vi "Initialize Hardware References.vi"(8 "error in (no error)":errorcluster caption="错误输入（无错误）", 11 "Hardware Resources in":T1={"PLC设置"={"端口选择"="COM3", "波特率"=0, "校检"=0, "数据位"=0}, "动作设置"={"自动跳法测试动作"={"夹紧"={"PLC指令"={"变量类型"=2, "PLC地址"="0", "16位/32位"=0, "写入数据(写入时有效)"=""}}, "分中"={}, "通油"={"打开主阀"={"变量类型"=2, "PLC地址"="0", "16位/32位"=0, "写入数据(写入时有效)"=""}, "打开电磁阀"={"变量类型"=2, "PLC地址"="0", "16位/32位"=0, "写入数据(写入时有效)"=""}}, "自动对中"={}, "内泄漏测试"={}, "压销"={"PLC指令"={"变量类型"=2, "PLC地址"="0", "16位/32位"=0, "写入数据(写入时有效)"=""}}}}} caption="硬件资源输入" {"动作设置"."自动跳法测试动作"."压销"."PLC指令"."16位/32位" items=["16bit", "32bit"]; "动作设置"."自动跳法测试动作"."压销"."PLC指令"."变量类型" items=["X", "Y", "M", "D"]; "动作设置"."自动跳法测试动作"."通油"."打开电磁阀"."16位/32位" items=["16bit", "32bit"]; "动作设置"."自动跳法测试动作"."通油"."打开电磁阀"."变量类型" items=["X", "Y", "M", "D"]; "动作设置"."自动跳法测试动作"."通油"."打开主阀"."16位/32位" items=["16bit", "32bit"]; "动作设置"."自动跳法测试动作"."通油"."打开主阀"."变量类型" items=["X", "Y", "M", "D"]; "动作设置"."自动跳法测试动作"."夹紧"."PLC指令"."16位/32位" items=["16bit", "32bit"]; "动作设置"."自动跳法测试动作"."夹紧"."PLC指令"."变量类型" items=["X", "Y", "M", "D"]; "PLC设置"."数据位" items=["7"=7, "8"=8]; "PLC设置"."校检" items=["无", "偶", "奇"]; "PLC设置"."波特率" items=["9600"=9600, "19200"=19200, "115200"=115200]}) -> (0 "error out":errorcluster caption="错误输出", 3 "Hardware Resources out":T1={"PLC设置"={"端口选择"="COM3", "波特率"=0, "校检"=0, "数据位"=0}, "动作设置"={"自动跳法测试动作"={"夹紧"={"PLC指令"={"变量类型"=2, "PLC地址"="0", "16位/32位"=0, "写入数据(写入时有效)"=""}}, "分中"={}, "通油"={"打开主阀"={"变量类型"=2, "PLC地址"="0", "16位/32位"=0, "写入数据(写入时有效)"=""}, "打开电磁阀"={"变量类型"=2, "PLC地址"="0", "16位/32位"=0, "写入数据(写入时有效)"=""}}, "自动对中"={}, "内泄漏测试"={}, "压销"={"PLC指令"={"变量类型"=2, "PLC地址"="0", "16位/32位"=0, "写入数据(写入时有效)"=""}}}}} caption="硬件资源输出" {"动作设置"."自动跳法测试动作"."压销"."PLC指令"."16位/32位" items=["16bit", "32bit"]; "动作设置"."自动跳法测试动作"."压销"."PLC指令"."变量类型" items=["X", "Y", "M", "D"]; "动作设置"."自动跳法测试动作"."通油"."打开电磁阀"."16位/32位" items=["16bit", "32bit"]; "动作设置"."自动跳法测试动作"."通油"."打开电磁阀"."变量类型" items=["X", "Y", "M", "D"]; "动作设置"."自动跳法测试动作"."通油"."打开主阀"."16位/32位" items=["16bit", "32bit"]; "动作设置"."自动跳法测试动作"."通油"."打开主阀"."变量类型" items=["X", "Y", "M", "D"]; "动作设置"."自动跳法测试动作"."夹紧"."PLC指令"."16位/32位" items=["16bit", "32bit"]; "动作设置"."自动跳法测试动作"."夹紧"."PLC指令"."变量类型" items=["X", "Y", "M", "D"]; "PLC设置"."数据位" items=["7"=7, "8"=8]; "PLC设置"."校检" items=["无", "偶", "奇"]; "PLC设置"."波特率" items=["9600"=9600, "19200"=19200, "115200"=115200]})   [LabVIEW 2015, in "Action.lvlib"]
doc: "初始化硬件引用。"
uses:
  Action.lvlib
  Hardware Configuration.ctl
  PLC/PLC.lvlib
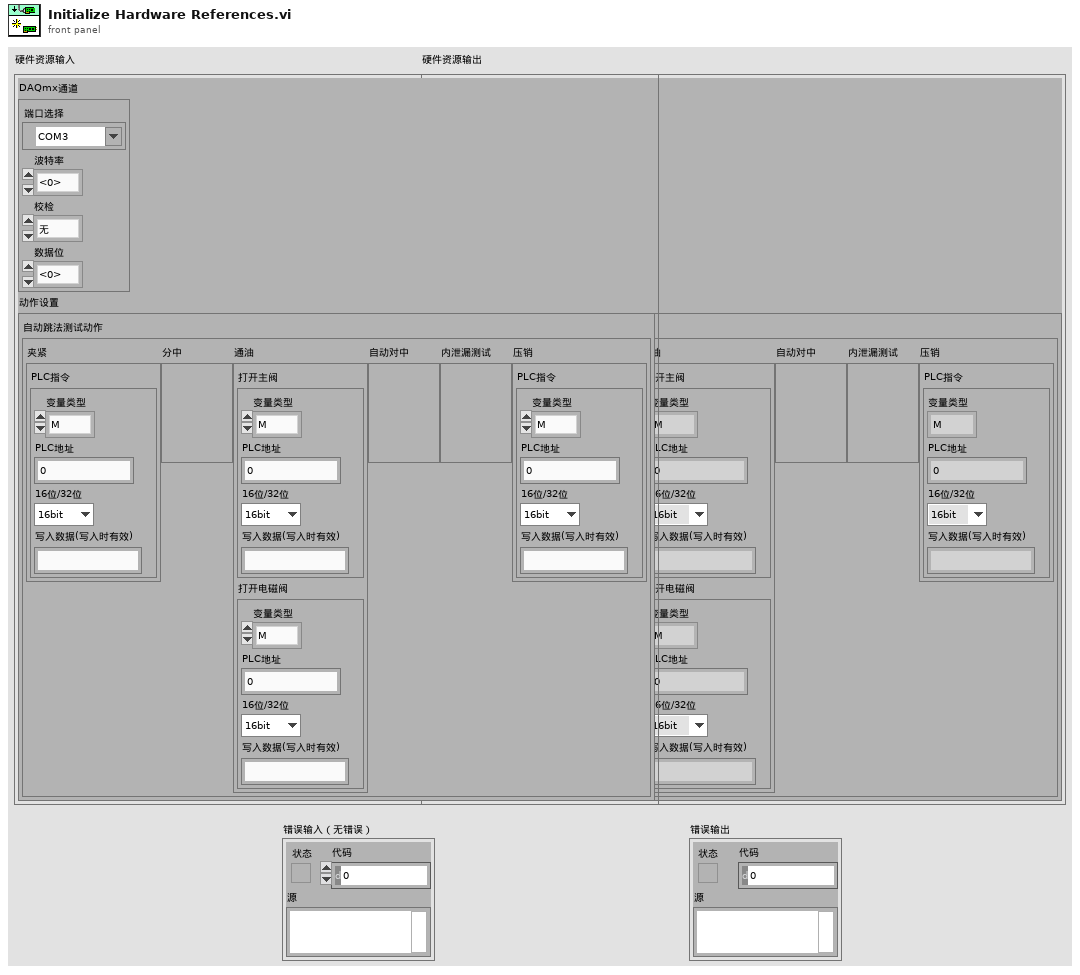
[diagram p1: front panel]
types:
  T1 = typedef "Action.lvlib/Hardware Configuration.ctl" = cluster{"PLC设置":T2, "动作设置":T3}
  T2 = typedef "PLC.lvlib/PLC设置.ctl" = cluster{"端口选择":refnum<visa-resource-name>, "波特率":u32, "校检":u32, "数据位":u32}
  T3 = typedef "Action.lvlib/动作设置.ctl" = cluster{"自动跳法测试动作":T4}
  T4 = typedef "Action.lvlib/自动调阀测试动作设置.ctl" = cluster{"夹紧":cluster{"PLC指令":T5}, "分中":cluster{}, "通油":cluster{"打开主阀":T5, "打开电磁阀":T5}, "自动对中":cluster{}, "内泄漏测试":cluster{}, "压销":cluster{"PLC指令":T5}}
  T5 = typedef "PLC.lvlib/PLC指令.ctl" = cluster{"变量类型":u32, "PLC地址":string, "16位/32位":u32, "写入数据(写入时有效)":string}
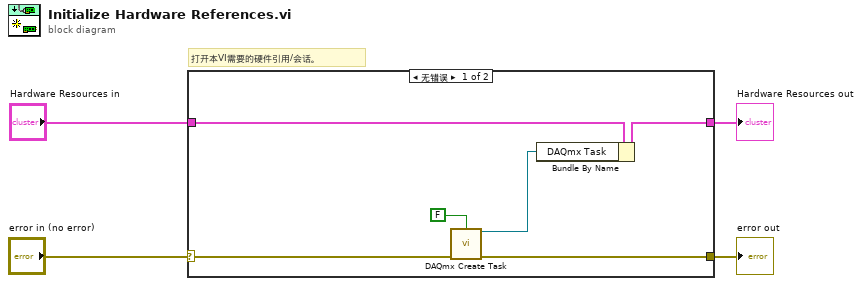
[diagram p0: block diagram]
diagram:
  # "打开本VI需要的硬件引用/会话。"
  n1 = case shown="无错误" "error in (no error)" {
    selector: "error in (no error)" -> [w7 w11]
    tunnel: [w5 w11] -> w3
    tunnel: "Hardware Resources in" -> [w9 w12]
    tunnel: [w10 w12] -> w1
    frame No Error {
      n2 = call <vilib>:"DAQmx Create Task.vi"("auto cleanup"=FALSE, "error in"=w7) -> ("task out"=w6:refnum<k21>, "error out"=w5:errorcluster)  [unwired: 12 in]
      n3 = Bundle By Name(cluster=w9, "DAQmx Task"=w6) -> (w10:T1)
    }
    frame Error {
    }
  }
  "Hardware Resources out" <- w1
  "error out" <- w3
